vi "Cluster to JSON File.vi"(8 "error in (no error)":errorcluster, 10 "Framework Configuration":T1, 11 "Framework Configuration in":refnum<class "Framework Configuration.lvclass">) -> (0 "error out":errorcluster, 3 "Framework Configuration out":refnum<class "Framework Configuration.lvclass">)   [LabVIEW 2017, in "Data Sharing Framework Engine.lvlib" / "Framework Configuration.lvclass"]
uses:
  Framework Configuration.lvclass
  Configuration/1.0.0/Public/Controls/DSF Engine Framework Configuration.ctl
  Configuration/1.0.0/Public/Controls/DSF Engine Plugin Configuration.ctl
  Configuration/1.0.0/Public/Controls/DSF Timing Info.ctl
  Configuration/1.0.0/Public/Controls/DSF Engine Transfer Group Configuration.ctl
  Configuration/1.0.0/Public/Controls/DSF Direction.ctl
  Configuration/1.0.0/Public/Controls/DSF Engine Transfer Configuration.ctl
  Configuration/1.0.0/Public/Controls/DSF Byte Order.ctl
  Configuration/1.0.0/Public/Controls/DSF Engine Channel Configuration.ctl
  Configuration/1.0.0/Public/Controls/DSF Data Type.ctl
  Configuration/1.0.0/Public/Controls/DSF Settings Info.ctl
  Framework Configuration.lvclass/Framework Configuration.ctl
  Configuration/1.0.0/DSF Configuration API.lvlib
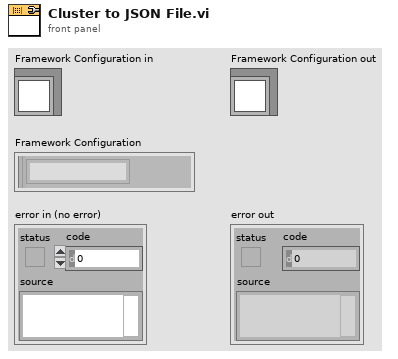
[diagram p1: front panel]
types:
  T1 = typedef "DSF Configuration API.lvlib/DSF Engine Framework Configuration.ctl" = cluster{"Plugins":T2[]}
  T2 = typedef "DSF Configuration API.lvlib/DSF Engine Plugin Configuration.ctl" = cluster{"name":string, "class":string, "cycle timing":T3, "Transfer Groups":T4[], "settings":T10}
  T3 = typedef "DSF Configuration API.lvlib/DSF Timing Info.ctl" = cluster{"priority":u64, "decimation":u64, "offset":u64}
  T4 = typedef "DSF Configuration API.lvlib/DSF Engine Transfer Group Configuration.ctl" = cluster{"name":string, "direction":T5, "cycle timing":T3, "Transfers":T6[], "settings":T10}
  T5 = typedef "DSF Configuration API.lvlib/DSF Direction.ctl" = enum8{"Tx", "Rx"}
  T6 = typedef "DSF Configuration API.lvlib/DSF Engine Transfer Configuration.ctl" = cluster{"name":string, "byte order":T7, "channel configurations":T8[], "settings":T10}
  T7 = typedef "DSF Configuration API.lvlib/DSF Byte Order.ctl" = enum8{"big-endian", "little-endian"}
  T8 = typedef "DSF Configuration API.lvlib/DSF Engine Channel Configuration.ctl" = cluster{"engine offset":u64, "name":string, "data type":T9, "count":u64, "buffer offset":u64, "settings":T10}
  T9 = typedef "DSF Configuration API.lvlib/DSF Data Type.ctl" = enum8{"Bool", "SGL", "DBL", "I8", "I16", "I32", "I64", "U8", "U16", "U32", "U64"}
  T10 = typedef "DSF Configuration API.lvlib/DSF Settings Info.ctl" = cluster{"key":string, "value":string}[]
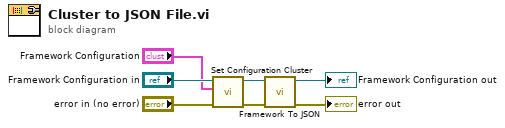
[diagram p0: block diagram]
diagram:
  n1 = call "Set Configuration Cluster.vi"("Framework Configuration"="Framework Configuration", "Framework Configuration in"="Framework Configuration in") -> ("Framework Configuration out"=w4:refnum<class "Framework Configuration.lvclass">)  [unwired: 9 in]
  n2 = call "Framework To JSON.vi"("error in (no error)"="error in (no error)", "Framework Configuration in"=w4) -> ("error out"=→"error out":errorcluster, "Framework Configuration out"=→"Framework Configuration out":refnum<class "Framework Configuration.lvclass">)  [unwired: 8 in]
